vi "Air to Methane Scale.vi"(9 "Air Flow (cfm)":dbl, 10 "Phi":dbl) -> (1 "Air Flow (cfm) out":dbl, 2 "Methane Flow (cfm)":dbl)   [LabVIEW 2013]
doc: "This sub-VI uses the desired equivalence ratio (phi) to scale the desired air flow (cfm) to desired\nmethane flow (cfm)."
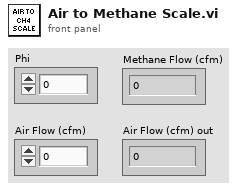
[diagram p1: front panel]
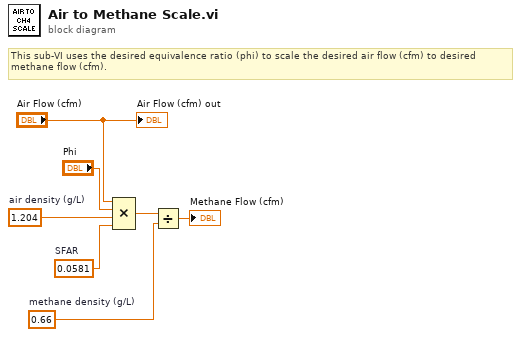
[diagram p0: block diagram]
diagram:
  w5 = 0.66  # methane density (g/L)
  w3 = 0.0581  # SFAR
  w2 = 1.204  # air density (g/L)
  # "This sub-VI uses the desired equivalence ratio (phi) to scale the desired air flow (cfm) to desired\nmethane flow (cfm)."
  n1 = Compound Arithmetic op=MULTIPLY("Air Flow (cfm)", "Phi", w2, w3) -> (w4:dbl)
  n2 = Divide(x=w4, y=w5) -> (x/y=→"Methane Flow (cfm)":dbl)
  "Air Flow (cfm) out" <- "Air Flow (cfm)"
